vi "buffer error.vi"(8 "error in":errorcluster, 11 "error buffer in":refnum<queue>) -> (3 "error buffer out":refnum<queue>)   [LabVIEW 2013, in "main engine.lvlib"]
uses:
  main engine/main engine.lvlib
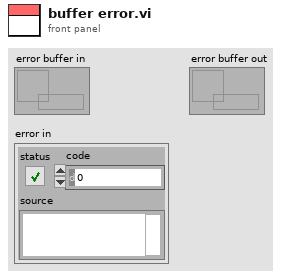
[diagram p1: front panel]
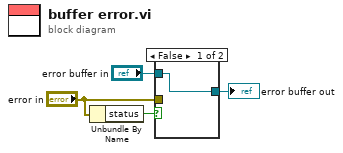
[diagram p0: block diagram]
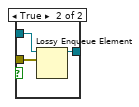
[diagram p2: hidden frame]
diagram:
  n1 = Unbundle By Name("error in") -> ("status"=w4:bool)
  n2 = case shown="False" w4 {
    tunnel: "error buffer in" -> [w5 w8]
    tunnel: "error in" -> [_ w7]
    tunnel: [w5 w6] -> w1
    frame False {
    }
    frame True {
      n3 = Lossy Enqueue Element(queue=w8, element=w7) -> (queue out=w6:refnum<queue>)  [unwired: 1 in, 3 out]
    }
  }
  "error buffer out" <- w1
